vi "editscenario Previous Scenarios.vi"(6 "User Information":T1, 8 "error in (no error)":errorcluster, 10 "sxScenarioId (\"\")":string, 11 "Connection Refnum":T2) -> (0 "error out":errorcluster, 2 "Previous SCENARIOS array":string, 3 "Connection Refnum":T2)   [LabVIEW 2011]
uses:
  SI.LIB/ODBC/SQL Controls/Connection Refnum.ctl
  server/database/Users/User Record.ctl
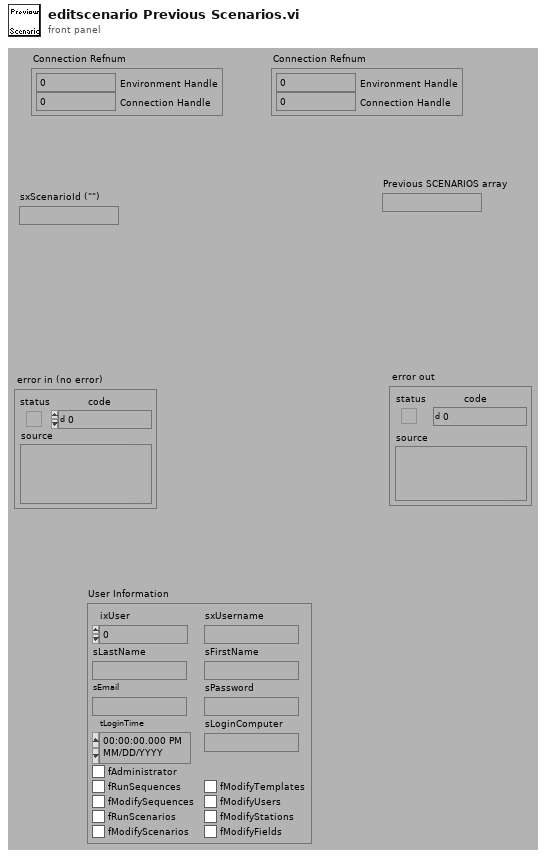
[diagram p1: front panel]
types:
  T1 = typedef "User Record.ctl" = cluster{"ixUser":i32, "sxUsername":string, "sLastName":string, "sFirstName":string, "sEmail":string, "sPassword":string, "tLoginTime":timestamp, "sLoginComputer":string, "fAdministrator":bool, "fRunSequences":bool, "fModifySequences":bool, "fRunScenarios":bool, "fModifyScenarios":bool, "fModifyTemplates":bool, "fModifyUsers":bool, "fModifyStations":bool, "fModifyFields":bool}
  T2 = typedef "Connection Refnum.ctl" = cluster{"Environment Handle":i32, "Connection Handle":i32}
  T3 = typedef "Scenario Record.ctl" = cluster{"ixScenario":i32, "tCreated":timestamp, "tModified":timestamp, "sxUsername":string, "sModifiedBy":string, "sxScenarioId":string, "sDescription":string, "sLogic":string, "sResultFieldsCSV":string, "sTemplatesCSV":string, "fAutoRunReports":bool, "fSortByTemplates":bool, "fCombinePDF":bool, "Conditions":T4[]}
  T4 = typedef "Condition Record.ctl" = cluster{"iConditionIndex":i32, "sxFieldId":string, "nOperator":T5, "sMatchValue":string}
  T5 = typedef "Condition Operators.ctl" = enum16{"equal (=)", "not equal (\\u2260)", "less than (<)", "less than or equal (\\u2264)", "greater than (>)", "greater than or equal (\\u2265)", "contains", "does not contain"}
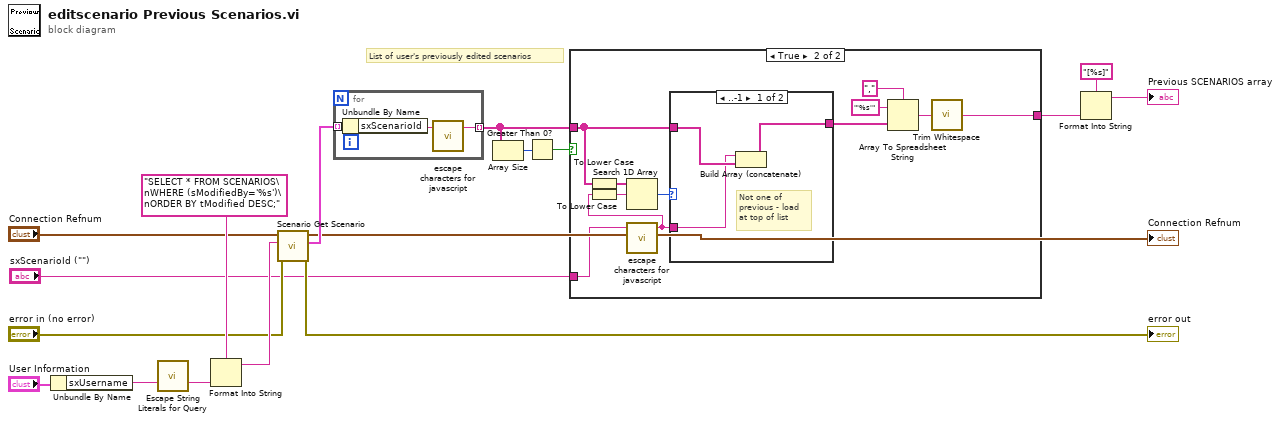
[diagram p0: block diagram]
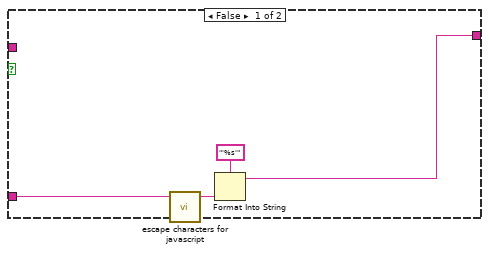
[diagram p2: hidden frame]
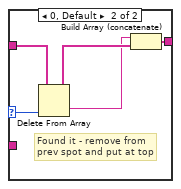
[diagram p3: hidden frame]
diagram:
  # "List of user's previously edited scenarios"
  n1 = Unbundle By Name("User Information") -> ("sxUsername"=w14:string)
  n2 = call "Escape String Literals for Query.vi"("String"=w14) -> ("escaped String"=w1:string)  [unwired: 1 in, 13 out]
  n3 = Format Into String(format string="SELECT * FROM SCENARIOS\nWHERE (sModifiedBy='%s')\nORDER BY tModified DESC;", w1) -> (resulting string=w16:string)  [unwired: 2 in, 1 out]
  n4 = call "Scenario Get Scenario.vi"("error in (no error)"="error in (no error)", "Query"=w16, "Connection Refnum"="Connection Refnum") -> ("error out"=→"error out":errorcluster, "Scenarios"=w15:T3[], "Connection Refnum"=→"Connection Refnum":T2)  [unwired: 6 out]
  n5 = for {
    tunnel: w15 -> [w20] mode=indexing
    tunnel: [w18] -> w3 mode=indexing
    n6 = Unbundle By Name(w20) -> ("sxScenarioId"=w19:string)
    n7 = call "escape characters for javascript.vi"("String (\"\")"=w19) -> ("escaped String"=w18:string)  [unwired: 4 out]
  }
  n8 = Array Size(array=w3) -> (size(s)=w7:i32)
  n9 = Greater Than 0?(x=w7) -> (x > 0?=w2:bool)
  n10 = case shown="True" w2 {
    tunnel: "sxScenarioId (\"\")" -> [w22 w29]
    tunnel: [w21 w27] -> w4
    tunnel: w3 -> [_ w26]
    frame False {
      n11 = call "escape characters for javascript.vi"("String (\"\")"=w22) -> ("escaped String"=w24:string)  [unwired: 4 out]
      n12 = Format Into String(format string="'%s'", w24) -> (resulting string=w21:string)  [unwired: 2 in, 1 out]
    }
    frame True {
      n13 = To Lower Case(string=w26) -> (all lower case string=w30:string[])
      n14 = call "escape characters for javascript.vi"("String (\"\")"=w29) -> ("escaped String"=w25:string)  [unwired: 4 out]
      n15 = To Lower Case(string=w25) -> (all lower case string=w32:string)
      n16 = Search 1D Array(1D array=w30, element=w32) -> (index of element=w31:i32)  [unwired: 1 out]
      n17 = case shown="..-1" w31 {
        selector: w31 -> [_ w42]
        tunnel: w26 -> [w38 w43]
        tunnel: w25 -> [w37 _]
        tunnel: [w36 w40] -> w28
        frame ..-1 {
          # "Not one of \nprevious - load\nat top of list"
          n18 = Build Array (concatenate)(w37, w38) -> (w36:string[])
        }
        frame 0, Default {
          # "Found it - remove from\nprev spot and put at top"
          n19 = Delete From Array(array=w43, index=w42) -> (deleted portion=w39:string, array with subset deleted=w41:string[])  [unwired: 1 in]
          n20 = Build Array (concatenate)(w39, w41) -> (w40:string[])
        }
      }
      n21 = Array To Spreadsheet String(delimiter (Tab)=",", array=w28, 3:"'%s'") -> (spreadsheet string=w33:string)
      n22 = call <vilib>:"Trim Whitespace.vi"("string"=w33) -> ("trimmed string"=w27:string)  [unwired: 1 in]
    }
  }
  n23 = Format Into String(format string="[%s]", w4) -> (resulting string=→"Previous SCENARIOS array":string)  [unwired: 2 in, 1 out]
